vi "StandardStateMachine 1.vi"() -> ()   [LabVIEW 2013]
doc: "使用该模板构建标准状态机设计模式。各状态执行代码并决定转移状态。将该设计模式与根据用户动作响应而执行代码的用户界面事件处理器模式相比较。同时将该设计模式与每段消息处理代码可以将零至多个新消息加入队列的队列消息处理器模式相比较。\n注：该模板的设计未遵守最新NI推荐的编程风格。请通过“创建项目”对话框（而不要采用该模板），创建基于项目的标准状态机模式的完整实现。"
uses:
  StateMachineStates 1.ctl
panel:
  in  "商店信息":cluster{"布尔":bool, "店名":string, "id":dbl}
  in  "数组":dbl[](array[numeric])
  in  "信息储存":string(tree)
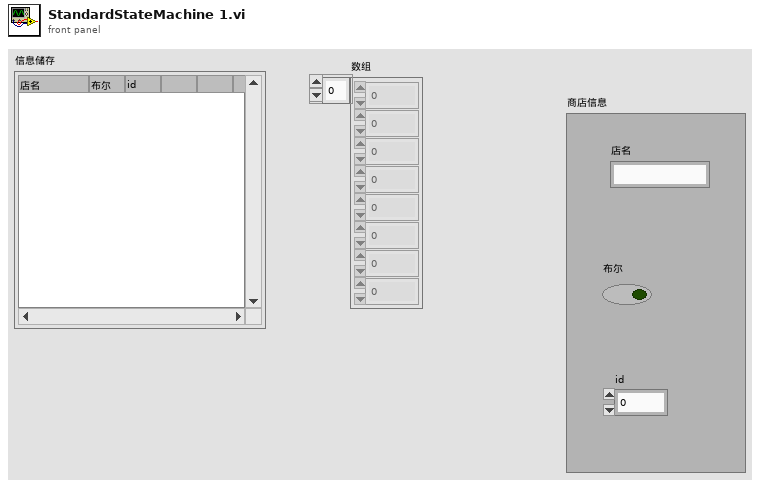
[diagram p1: front panel]
types:
  T1 = typedef "StateMachineStates 1.ctl" = enum16{"Initialize", "Stop"}
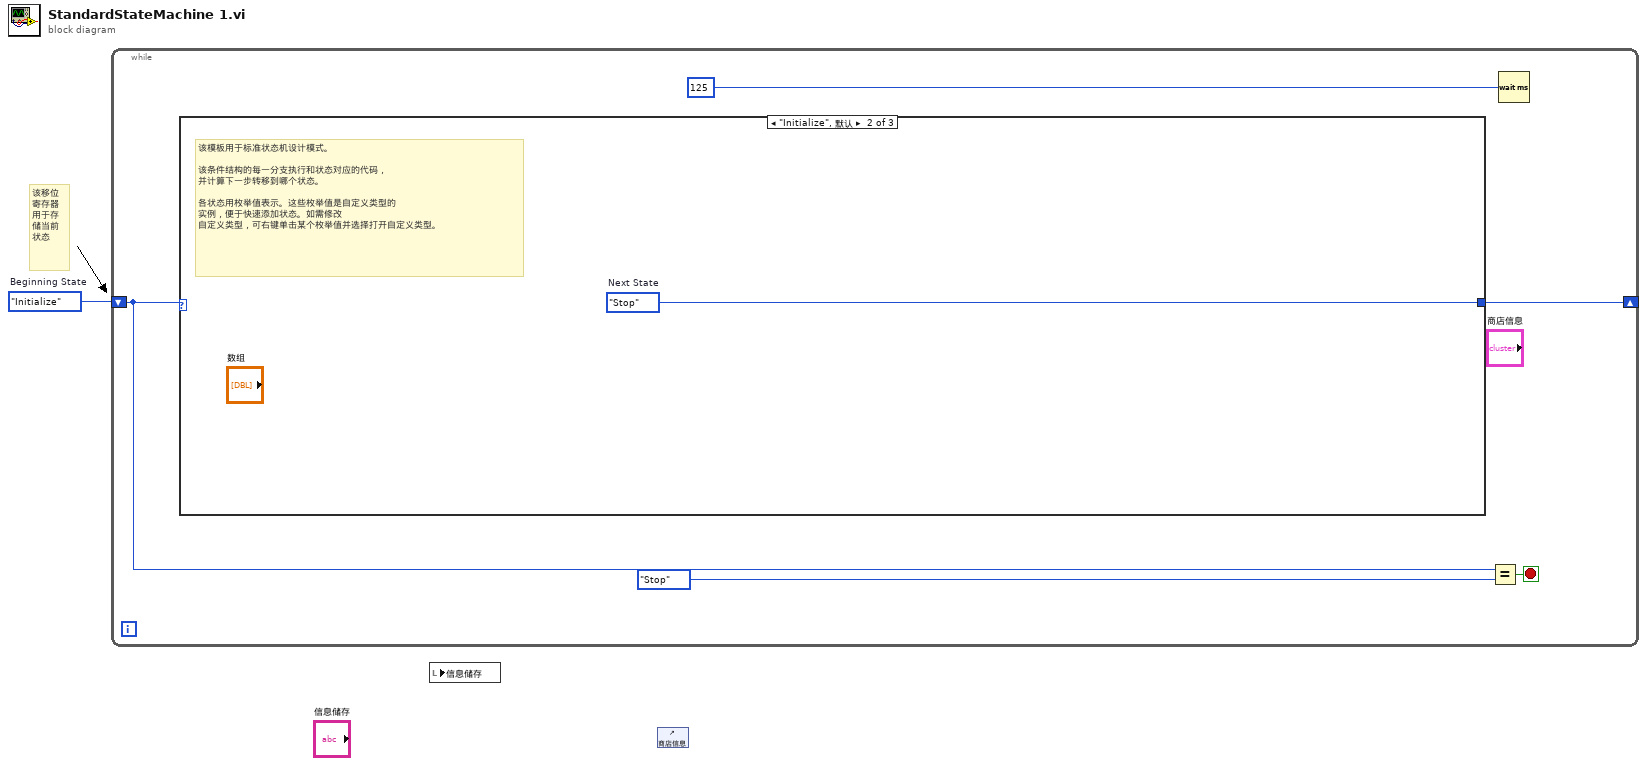
[diagram p0: block diagram]
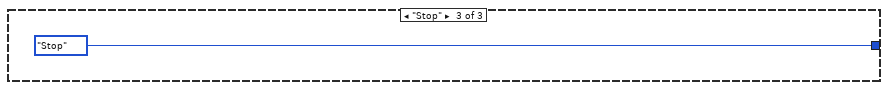
[diagram p3: hidden frame]
diagram:
  w1 = StateMachineStates_1."Initialize"  # Beginning State
  # "该移位\n寄存器\n用于存\n储当前\n状态"
  n1 = while {
    shift-right: [w3] -> _
    shift-left: w1 -> [w4]
    stop <- w6 stop-if-true
    n2 = case shown="\"Initialize\", 默认" w4 {
      tunnel: [_ w7 StateMachineStates_1."Stop" ("Next State")] -> w3
      frame "Initialize" {
      }
      frame "Initialize", Default {
        w7 = StateMachineStates_1."Stop"  # Next State
        # "该模板用于标准状态机设计模式。\n\n该条件结构的每一分支执行和状态对应的代码，\n并计算下一步转移到哪个状态。\n\n各状态用枚举值表示。这些枚举值是自定义类型的\n实例，便于快速添加状态。如需修改\n自定义类型，可右键单击某个枚举值并选择打开自定义类型。"
      }
      frame "Stop" {
      }
    }
    n3 = Equal?(x=w4, y=StateMachineStates_1."Stop" ("States")) -> (x = y?=w6:bool)
    n4 = Wait (ms)(milliseconds to wait=u32 125) -> ()  [unwired: 1 out]
  }
  n5 = local read "信息储存"() -> ()  [unwired: 1 in]
  n6 = control-ref of="商店信息"() -> ()  [unwired: 1 out]
